vi "Send.vi"(10 "String Indicator":string) -> (3 "String Indicator Ref out":refnum<class "String Indicator Ref.lvclass">)   [LabVIEW 2021, in "String Indicator Ref.lvlib" / "String Indicator Ref.lvclass"]
uses:
  String Indicator Ref.lvclass
  String Indicator Ref.lvclass/String Indicator Ref.ctl
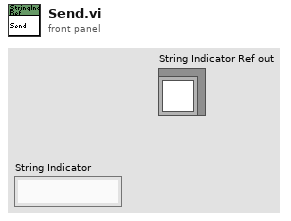
[diagram p1: front panel]
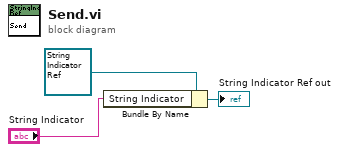
[diagram p0: block diagram]
diagram:
  n1 = Bundle By Name(cluster=refnum<class "String Indicator Ref.lvclass"> refnum ("String Indicator Ref out"), "String Indicator"="String Indicator") -> (→"String Indicator Ref out":refnum<class "String Indicator Ref.lvclass">)
